vi "LightningPID.vi"(8 "PID Settings":T1, 9 "Reset":bool, 10 "Position":dbl, 11 "Set Point":dbl) -> (3 "Output":dbl)   [LabVIEW 2014]
uses:
  LightningPID Settings.ctl
panel:
  out "dBase":dbl(graph)
  out "iState":dbl(graph)
  out "dBase":dbl
  out "iState":dbl
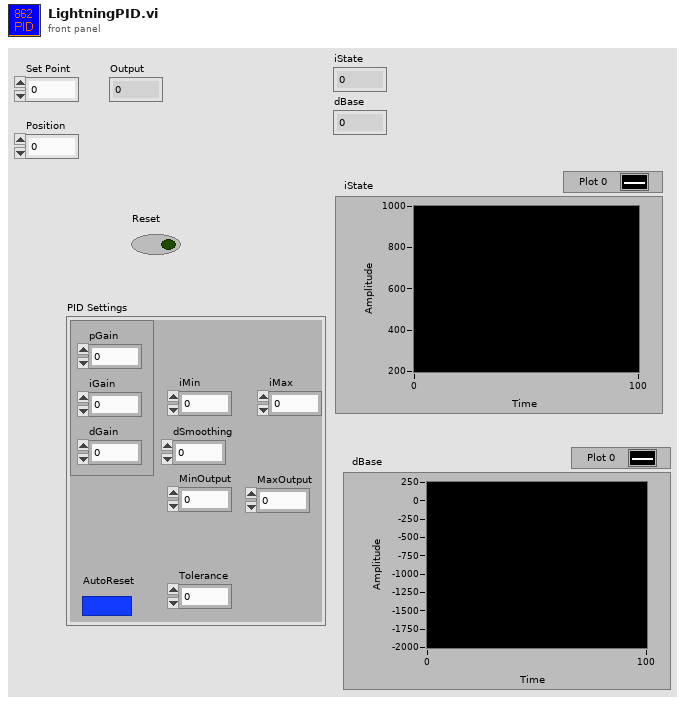
[diagram p1: front panel]
types:
  T1 = typedef "LightningPID Settings.ctl" = cluster{"iMax":dbl, "iMin":dbl, "iGain":dbl, "pGain":dbl, "dGain":dbl, "MaxOutput":dbl, "MinOutput":dbl, "AutoReset":bool, "Tolerance":dbl, "dSmoothing":dbl}
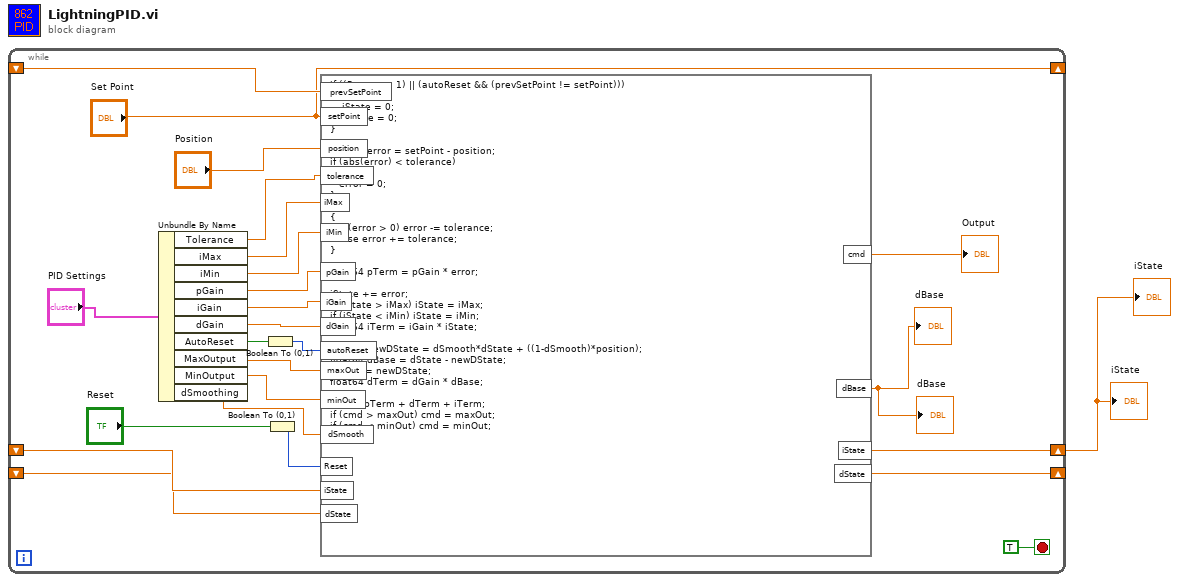
[diagram p0: block diagram]
diagram:
  n1 = while {
    shift-right: [w19] -> w1
    shift-left: _ -> [w17]
    shift-right: [w18] -> _
    shift-left: _ -> [w16]
    shift-right: ["Set Point"] -> _
    shift-left: _ -> [w15]
    stop <- TRUE stop-if-true
    n2 = Unbundle By Name("PID Settings") -> ("Tolerance"=w4:dbl, "iMax"=w24:dbl, "iMin"=w6:dbl, "pGain"=w23:dbl, "iGain"=w22:dbl, "dGain"=w21:dbl, "AutoReset"=w13:bool, "MaxOutput"=w8:dbl, "MinOutput"=w7:dbl, "dSmoothing"=w3:dbl)
    n3 = Boolean To (0,1)(Boolean=w13) -> (0, 1=w14:i16)
    n4 = Boolean To (0,1)(Boolean="Reset") -> (0, 1=w12:i16)
    n5 = formula code="if ((Reset == 1) || (autoReset && (prevSetPoint != setPoint)))\n{\n    iState = 0;\n    dState = 0;\n}\n\nfloat64 error = setPoint - position;\nif (abs(error) < tolerance) \n{\n   error = 0;\n}\nelse\n{\n   if (error > 0) error -= tolerance;\n   else error += tolerance;\n}\n\nfloat64 pTerm = pGain * error;\n\niState += error;\nif (iState > iMax) iState = iMax;\nif (iState < iMin) iState = iMin;\nfloat64 iTerm = iGain * iState;\n\nfloat64 newDState = dSmooth*dState + ((1-dSmooth)*position);\nfloat64 dBase = dState - newDState;\ndState = newDState;\nfloat64 dTerm = dGain * dBase;\n\ncmd = pTerm + dTerm + iTerm;\nif (cmd > maxOut) cmd = maxOut;\nif (cmd < minOut) cmd = minOut;"("position"="Position", "dState"=w16, "iState"=w17, "pGain"=w23, "iGain"=w22, "dGain"=w21, "iMax"=w24, "iMin"=w6, "Reset"=w12, "prevSetPoint"=w15, "autoReset"=w14, "setPoint"="Set Point", "maxOut"=w8, "minOut"=w7, "tolerance"=w4, "dSmooth"=w3) -> ("cmd"=→"Output":dbl, "iState"=w19:dbl, "dState"=w18:dbl, "dBase"=→"dBase" →"dBase":dbl)
  }
  "iState" <- w1
  "iState" <- w1
